vi "Read-Execute-Print-Loop with a Raspberry Pi.vi"() -> ()   [LabVIEW 2018]
doc: "Demonstrates an implementation of Read-Evaluate-Print-Loop (REPL) with a Raspberry Pi as the remote SSH server. This is similar to connecting to a Raspberry Pi through a shell or terminal with a SSH client command line interface or PuTTY on Windows. The remote SSH server could also be a CompactRIO with the remote SSH server enabled."
uses:
  Toolkit/Channel/Type Definitions/Modes.ctl
  Toolkit/Channel/Channel.lvclass/Channel.ctl
  Toolkit/Session/Session.lvclass/Session.ctl
  Toolkit/SSH/SSH.lvclass/SSH.ctl
  Toolkit/Session/Utility/Read Shared Library.vi
  Toolkit/SSH/Utility/Read Shared Library.vi
  Toolkit/Session/Support/Create from SSH.vi
  Toolkit/Session/Support/Password Authentication.vi
  Toolkit/Channel/Support/Create from Session.vi
  Toolkit/Support/Check Status.vi
  Toolkit/Channel/Support/Destroy to Session.vi
  Toolkit/Session/Support/Destroy to SSH.vi
  Toolkit/SSH/SSH.lvclass
  Toolkit/Session/Session.lvclass
  Toolkit/Channel/Channel.lvclass
panel:
  out "Last Command":string
  out "Read Buffer":string="1. Run this VI\n2. Enter Password\n3. Type a command\n4. Press ENTER or RETURN\n5. Observe the content of this indicator\n6. Close the VI to safely exit"
  in  "Command":string
  in  "Raspberry Pi Address":string="raspberrypi.local"
  in  "Password":string
  in  "Username":string="pi"
  # "Overview: Demonstrates simultaneous reading and writing with a SSH channel to a Raspberry Pi\nInstructions:\n1. Run this VI.\n2. Change the Raspberry Pi Address from the mDNS default to another mDNS or the IP address of the Raspberry Pi if needed.\n3. Change the username from the default Raspberry Pi user if needed.\n4. Enter the password for the Raspberry Pi user and press ENTER or RETURN\n5. Observe the Read Buffer's content.\n6. Enter a command.\n7. Press ENTER or RETURN\n8. Observe the read Buffer's content.\n9. Close the VI"
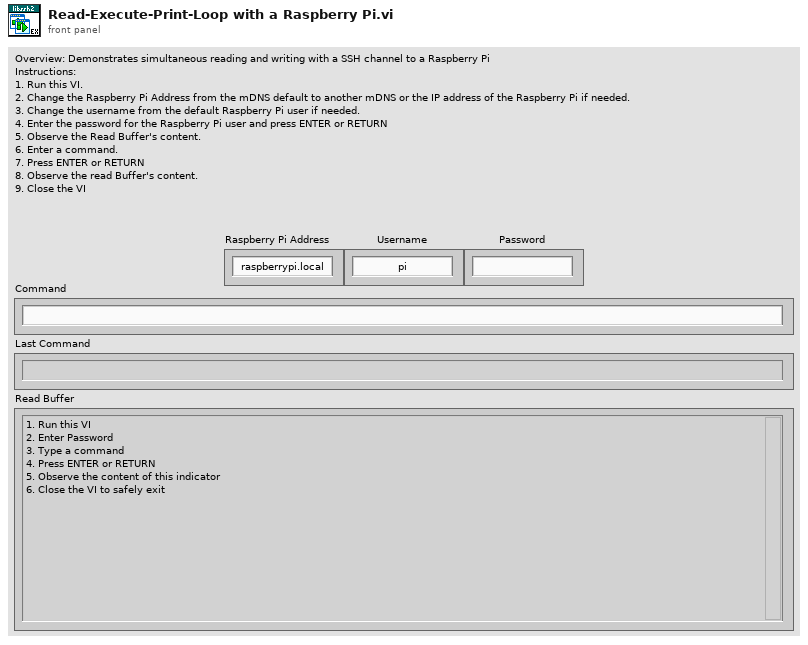
[diagram p1: front panel]
types:
  T1 = typedef "Toolkit.lvlib/Channel.lvclass/Modes.ctl" = i32
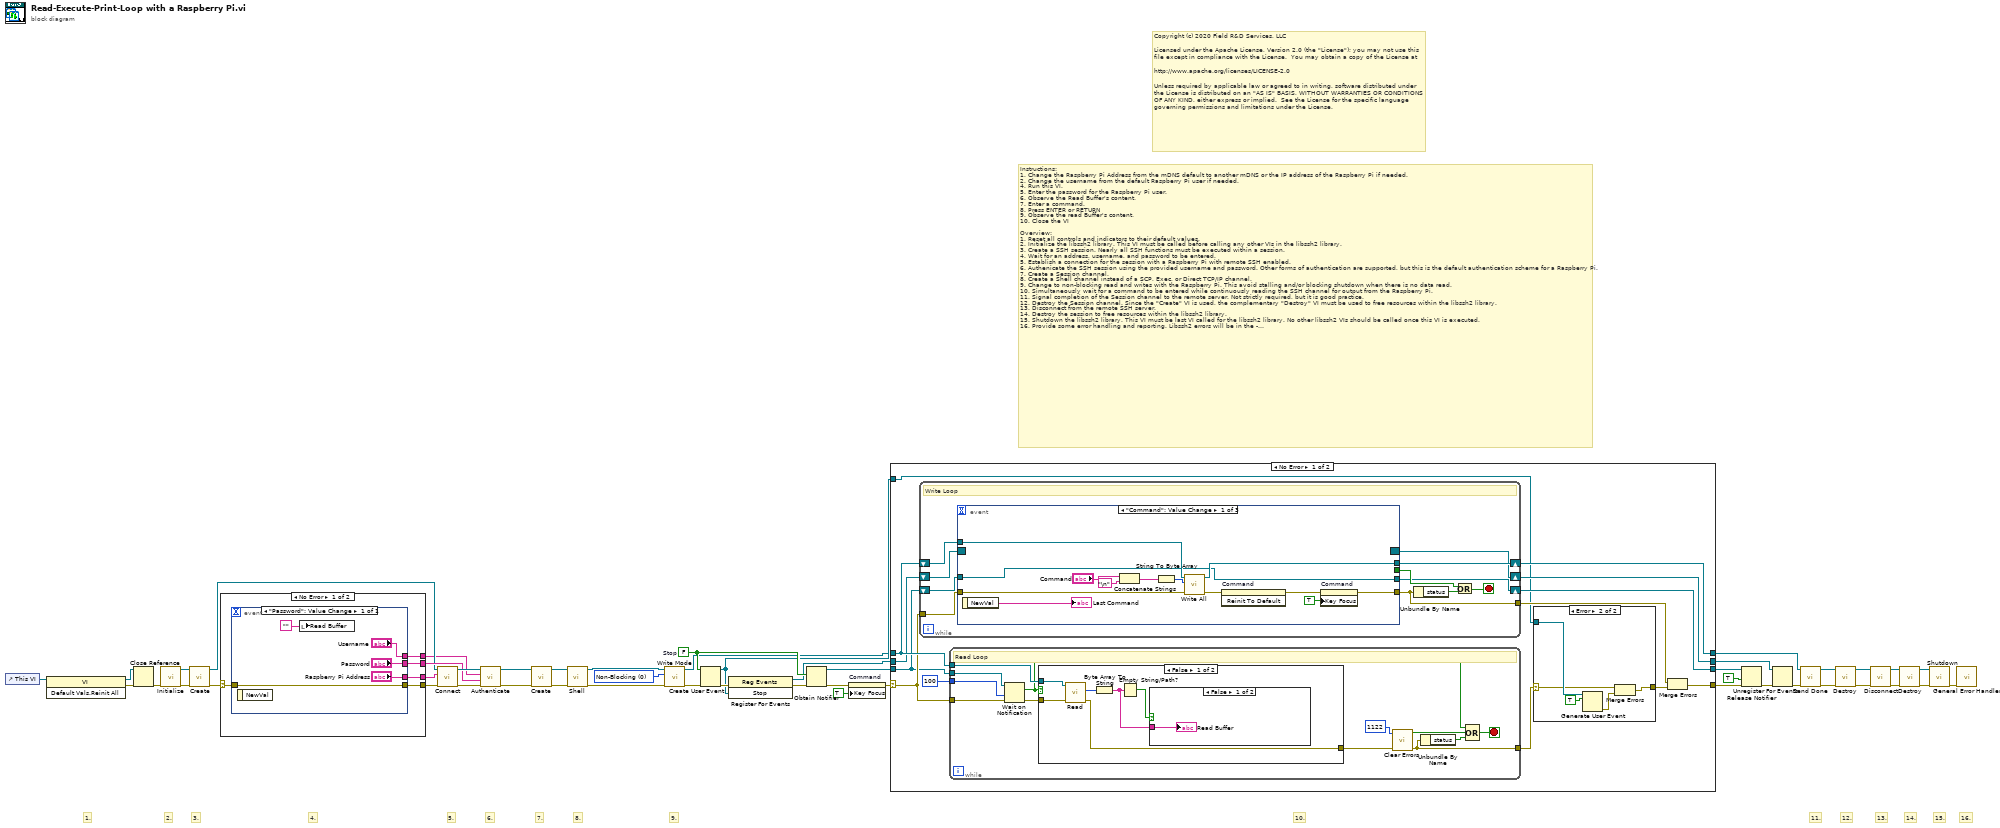
[diagram p0: block diagram]
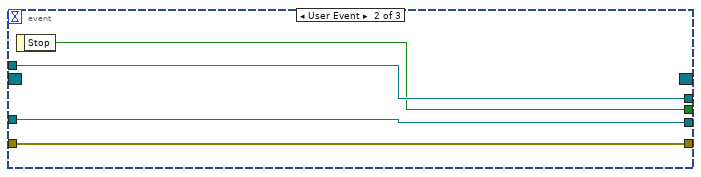
[diagram p3: hidden frame]
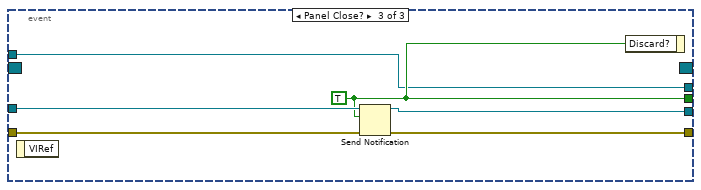
[diagram p4: hidden frame]
diagram:
  w3 = T1 0 items=["Non-Blocking", "Blocking"] ("Mode")
  w23 = FALSE  # Stop
  # "4."
  # "16."
  # "15."
  # "14."
  # "13."
  # "12."
  # "11."
  # "10."
  # "9."
  # "8."
  # "7."
  # "6."
  # "5."
  # "3."
  # "2."
  # "1."
  # "Instructions:\n1. Change the Raspberry Pi Address from the mDNS default to another mDNS or the IP address of the Raspberry Pi if needed.\n2. Change the username from the default Raspberry Pi user if needed.\n4. Run this VI.\n5. Enter the password for the Raspberry Pi user.\n6. Observe the Read Buffer's content.\n7. Enter a command.\n8. Press ENTER or RETURN\n9. Observe the read Buffer's content.\n10. Close the VI\n\nOverview:\n1. Reset all controls and indicators to their default values.\n2. Initialize the libssh2 library. This VI must be called before calling any other VIs in the libssh2 library.\n3. Create a SSH session. Nearly all SSH functions must be executed within a session.\n4. Wait for an address, username, and password to be entered. \n5. Establish a connection for the session with a Raspberry Pi with remote SSH enabled.\n6. Authenicate the SSH session using the provided username and password. Other forms of authentication are supported, but this is the default authentication scheme for a Raspberry Pi. \n7. Create a Session channel.\n8. Create a Shell channel instead of a SCP, Exec, or Direct TCP/IP channel.\n9. Change to non-blocking read and writes with the Raspberry Pi. This avoid stalling and/or blocking shutdown when there is no data read.\n10. Simultaneously wait for a command to be entered while continuously reading the SSH channel for output from the Raspberry Pi.\n11. Signal completion of the Session channel to the remote server. Not strictly required, but it is good practice. \n12. Destroy the Session channel. Since the \"Create\" VI is used, the complementary \"Destroy\" VI must be used to free resources within the libssh2 library. \n13. Disconnect from the remote SSH server.\n14. Destroy the session to free resources within the libssh2 library.\n15. Shutdown the libssh2 library. This VI must be last VI called for the libssh2 library. No other libssh2 VIs should be called once this VI is executed.\n16. Provide some error handling and reporting. Libssh2 errors will be in the -8100 range."
  # "Copyright (c) 2020 Field R&D Services, LLC\n\nLicensed under the Apache License, Version 2.0 (the \"License\"); you may not use this file except in compliance with the License.  You may obtain a copy of the License at\n\nhttp://www.apache.org/licenses/LICENSE-2.0\n\nUnless required by applicable law or agreed to in writing, software distributed under the License is distributed on an \"AS IS\" BASIS, WITHOUT WARRANTIES OR CONDITIONS OF ANY KIND, either express or implied.  See the License for the specific language governing permissions and limitations under the License."
  n1 = control-ref of="This VI"() -> (w27:refnum<vi>)
  n2 = invoke class="VI" method="Default Vals.Reinit All"(reference=w27) -> (reference out=w26:refnum<vi>, error out=w25:errorcluster)  [unwired: 2 in, 1 out]
  n3 = Close Reference(reference=w26, error in (no error)=w25) -> (error out=w24:errorcluster)
  n4 = call "Initialize.vi"("Error In"=w24) -> ("Error Out"=w47:errorcluster, "SSH"=w48:refnum<class "SSH.lvclass">)  [unwired: 9 in]
  n5 = call-poly "Create.vi"("Error In"=w47, "SSH"=w48) -> ("Error Out"=w15:errorcluster, "Sesssion"=w14:refnum<class "Session.lvclass">)  [unwired: 8 in]
  n6 = case shown="No Error" w15 {
    selector: w15 -> [w52 w59]
    tunnel: [w53 _] -> w38
    tunnel: [w51 w59] -> w13
    tunnel: [w50 _] -> w11
    tunnel: [w49 _] -> w10
    frame No Error {
      n7 = event shown="[0] \"Password\": Value Change" {
        selector: _ -> [_]
        dyn-events: _ -> [_]
        timeout: _ -> [_]
        tunnel: ["Password"] -> w53
        tunnel: w52 -> [w57]
        tunnel: [w57] -> w51
        tunnel: ["Raspberry Pi Address"] -> w50
        tunnel: ["Username"] -> w49
        event "Password": Value Change {
          n8 = event-data() -> ()  [unwired: 1 in, 1 out]
          n9 = local write "Read Buffer"("") -> ()
        }
      }
    }
    frame Error {
    }
  }
  n10 = call "Connect.vi"("Error In"=w13, "Address"=w11, "Session In"=w14) -> ("Error Out"=w12:errorcluster, "Sesssion Out"=w46:refnum<class "Session.lvclass">)  [unwired: 7 in]
  n11 = call-poly "Authenticate.vi"("Error In"=w12, "Password"=w38, "Username"=w10, "Session In"=w46) -> ("Error Out"=w44:errorcluster, "Sesssion Out"=w45:refnum<class "Session.lvclass">)  [unwired: 6 in]
  n12 = call-poly "Create.vi"("Error In"=w44, "Session"=w45) -> ("Error Out"=w4:errorcluster, "Channel"=w5:refnum<class "Channel.lvclass">)  [unwired: 8 in]
  n13 = call "Shell.vi"("Error In"=w4, "Channel In"=w5) -> ("Error Out"=w6:errorcluster, "Channel Out"=w9:refnum<class "Channel.lvclass">)  [unwired: 8 in]
  n14 = call "Write Mode.vi"("Error In"=w6, "Mode"=w3, "Channel In"=w9) -> ("Error Out"=w7:errorcluster, "Channel Out"=w8:refnum<class "Channel.lvclass">)  [unwired: 7 in]
  n15 = Create User Event(user event datatype=w23, error in=w7) -> (user event=w16:refnum<user-event>, error out=w22:errorcluster)
  n16 = register-events(error in=w22, w16) -> (reference out=w20:refnum<event-registration>, error out=w21:errorcluster)  [unwired: 1 in]
  n17 = Obtain Notifier(notification data type=w23, error in (no error)=w21) -> (notifier out=w31:refnum<notifier>, error out=w32:errorcluster)  [unwired: 2 in, 1 out]
  n18 = property on="Command" class="Str"(error in=w32, "Key Focus"=TRUE) -> (error out=w2:errorcluster)  [unwired: 1 in, 1 out]
  n19 = case shown="No Error" w2 {
    selector: w2 -> [w71 w135]
    tunnel: w8 -> [w72 w136]
    tunnel: [w70 w136] -> w36
    tunnel: [w68 w135] -> w30
    tunnel: w31 -> [w67 w134]
    tunnel: [w66 w134] -> w29
    tunnel: w20 -> [w65 w133]
    tunnel: [w64 w133] -> w17
    tunnel: w16 -> [w61 _]
    frame No Error {
      n20 = while {
        tunnel: w71 -> [w83]
        tunnel: [w79] -> w69
        shift-right: [w81] -> w70
        shift-left: w72 -> [w82]
        shift-right: [w75] -> w66
        shift-left: w67 -> [w76]
        shift-right: [w73] -> w64
        shift-left: w65 -> [w74]
        stop <- w77 stop-if-true
        # "Write Loop"
        n21 = event shown="[0] \"Command\": Value Change" {
          selector: w74 -> [_ _ _]
          dyn-events: [_ _ _] -> w73
          timeout: _ -> [_ _ _]
          tunnel: w83 -> [w96 w99 w102]
          tunnel: [w84 w99 w105] -> w79
          tunnel: w82 -> [w95 w98 w101]
          tunnel: [w93 w98 w101] -> w81
          tunnel: [_ w97 w103] -> w80
          tunnel: w76 -> [w92 w100 w106]
          tunnel: [w92 w100 w104] -> w75
          event "Command": Value Change {
            n22 = event-data() -> ("NewVal"=→"Last Command":string)  [unwired: 1 in]
            n23 = Concatenate Strings("Command", "\n") -> (w91:string)
            n24 = String To Byte Array(string=w91) -> (unsigned byte array=w94:u8[])
            n25 = call "Write All.vi"("Error In"=w96, "Data"=w94, "Channel In"=w95) -> ("Error Out"=w87:errorcluster, "Channel Out"=w93:refnum<class "Channel.lvclass">)  [unwired: 5 in, 2 out]
            n26 = invoke on="Command" class="Str" method="Reinit To Default"(error in=w87) -> (error out=w85:errorcluster)  [unwired: 2 in, 2 out]
            n27 = property on="Command" class="Str"(error in=w85, "Key Focus"=TRUE) -> (error out=w84:errorcluster)  [unwired: 1 in, 1 out]
          }
          event User Event {
            n28 = event-data() -> ("Stop"=w97:bool)  [unwired: 1 in]
          }
          event Panel Close? {
            w103 = TRUE ("Discard?")
            n29 = event-data() -> ()  [unwired: 1 in, 1 out]
            n30 = Send Notification(notification=w103, notifier=w106, error in (no error)=w102) -> (notifier out=w104:refnum<notifier>, error out=w105:errorcluster)
            n31 = event-data("Discard?"=w103) -> ()  [unwired: 1 in, 1 out]
          }
        }
        n32 = Unbundle By Name(w79) -> ("status"=w78:bool)
        n33 = Or(x=w80, y=w78) -> (x .or. y?=w77:bool)
      }
      n34 = while {
        tunnel: w72 -> [w118]
        tunnel: w71 -> [w117]
        tunnel: [w108] -> w63
        tunnel: w67 -> [w115]
        tunnel: 100 ("timeout in ms (-1)") -> [w107]
        stop <- w110 stop-if-true
        # "Read Loop"
        n35 = Wait on Notification(notifier=w115, timeout in ms (-1)=w107, error in (no error)=w117) -> (notification=w109:bool, error out=w116:errorcluster)  [unwired: 1 in, 2 out]
        n36 = case shown="False" w109 {
          tunnel: w118 -> [w124 _]
          tunnel: w116 -> [w122 w126]
          tunnel: [w121 w126] -> w114
          frame False {
            n37 = call "Read.vi"("Error In"=w122, "Channel In"=w124) -> ("Error Out"=w121:errorcluster, "Data"=w123:u8[])  [unwired: 7 in, 1 out]
            n38 = Byte Array To String(unsigned byte array=w123) -> (string=w120:string)
            n39 = Empty String/Path?(string/path=w120) -> (empty?=w119:bool)
            n40 = case shown="False" w119 {
              tunnel: w120 -> [w125 _]
              frame False {
                "Read Buffer" <- w125
              }
              frame True {
              }
            }
          }
          frame True {
          }
        }
        n41 = call <vilib>:"Clear Errors.vi"("error in (no error)"=w114, "specific error code to clear (0: all)"=1122) -> ("error out"=w108:errorcluster, "specific error cleared?"=w112:bool)  [unwired: 4 in]
        n42 = Unbundle By Name(w108) -> ("status"=w111:bool)
        n43 = Compound Arithmetic op=OR(w109, w112, w111) -> (w110:bool)
      }
      n44 = case shown="Error" w63 {
        selector: w63 -> [w127 w130]
        tunnel: [w127 w128] -> w62
        tunnel: w61 -> [_ w132]
        frame No Error {
        }
        frame Error {
          n45 = Generate User Event(user event=w132, event data cluster=TRUE ("event data")) -> (error out=w129:errorcluster)  [unwired: 2 in, 1 out]
          n46 = Merge Errors(w130, w129) -> (w128:errorcluster)
        }
      }
      n47 = Merge Errors(w69, w62) -> (w68:errorcluster)
    }
    frame Error {
    }
  }
  n48 = Release Notifier(notifier=w29, force destroy? (F)=TRUE, error in (no error)=w30) -> (error out=w19:errorcluster)  [unwired: 2 out]
  n49 = Unregister For Events(event registration refnum=w17, error in=w19) -> (error out=w18:errorcluster)
  n50 = call "Send Done.vi"("Error In"=w18, "Channel In"=w36) -> ("Error Out"=w33:errorcluster, "Channel Out"=w35:refnum<class "Channel.lvclass">)  [unwired: 8 in]
  n51 = call-poly "Destroy.vi"("Error In"=w33, "Channel"=w35) -> ("Error Out"=w43:errorcluster, "Session"=w34:refnum<class "Session.lvclass">)  [unwired: 8 in]
  n52 = call "Disconnect.vi"("Error In"=w43, "Session In"=w34) -> ("Error Out"=w41:errorcluster, "Sesssion Out"=w42:refnum<class "Session.lvclass">)  [unwired: 8 in]
  n53 = call-poly "Destroy.vi"("Error In"=w41, "Session"=w42) -> ("Error Out"=w39:errorcluster, "SSH"=w40:refnum<class "SSH.lvclass">)  [unwired: 8 in]
  n54 = call "Shutdown.vi"("Error In"=w39, "SSH"=w40) -> ("Error Out"=w37:errorcluster)  [unwired: 9 in]
  n55 = call <vilib>:"General Error Handler.vi"("error in (no error)"=w37) -> ()  [unwired: 10 in, 5 out]
